vi "Previous to Target Version.vi"(1 "Previous Version":T1) -> (0 "Target Version":string)   [LabVIEW 2017, in "Scripts.lvlib"]
doc: "Converts the LabVIEW Previous Version enum to a Target Version string with format \"Major.Minor\". For example, 2015 is converted to 15.0."
uses:
  Scripts.lvlib
  Controls/LabVIEW Versions.ctl
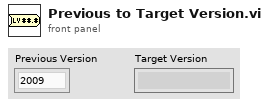
[diagram p1: front panel]
types:
  T1 = typedef "Scripts.lvlib/LabVIEW Versions.ctl" = enum16{"2009", "2010", "2011", "2012", "2013", "2014", "2015", "2016", "2017", "2018"}
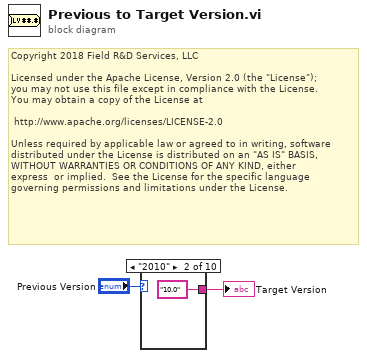
[diagram p0: block diagram]
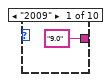
[diagram p2: hidden frame]
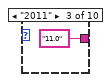
[diagram p3: hidden frame]
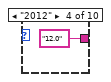
[diagram p4: hidden frame]
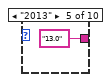
[diagram p5: hidden frame]
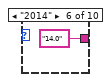
[diagram p6: hidden frame]
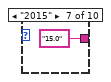
[diagram p7: hidden frame]
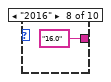
[diagram p8: hidden frame]
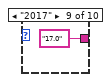
[diagram p9: hidden frame]
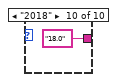
[diagram p10: hidden frame]
diagram:
  # "Copyright 2018 Field R&D Services, LLC\n\nLicensed under the Apache License, Version 2.0 (the \"License\");\nyou may not use this file except in compliance with the License.\nYou may obtain a copy of the License at\n\n\thttp://www.apache.org/licenses/LICENSE-2.0\n\nUnless required by applicable law or agreed to in writing, software\ndistributed under the License is distributed on an \"AS IS\" BASIS,\nWITHOUT WARRANTIES OR CONDITIONS OF ANY KIND, either \nexpress  or implied.  See the License for the specific language \ngoverning permissions and limitations under the License."
  n1 = case shown="\"2010\"" "Previous Version" {
    tunnel: ["9.0" "10.0" "11.0" "12.0" "13.0" "14.0" "15.0" "16.0" "17.0" "18.0"] -> w2
    frame "2009" {
    }
    frame "2010" {
    }
    frame "2011" {
    }
    frame "2012" {
    }
    frame "2013" {
    }
    frame "2014" {
    }
    frame "2015" {
    }
    frame "2016" {
    }
    frame "2017" {
    }
    frame "2018" {
    }
  }
  "Target Version" <- w2
